vi "readblink.vi"() -> ()   [LabVIEW 2014]
uses:
  <vilib>/LabVIEW Interface for Arduino/Type Defs/Board Type.ctl
  <vilib>/addons/_Advanced Signal Processing/NI_AdvSigProcWA.lvlib
  <vilib>/LabVIEW Interface for Arduino/LabVIEW Interface for Arduino.lvlib
panel:
  in  "stop":bool
  out "Filtered Signal 4":waveform(dbl)(graph) caption="Filtered Signal"
  out "Boolean":bool
  out "Result":dynamicdata(graph)
  out "Filtered Signal 3":dynamicdata(graph) caption="Filtered Signal"
  out "Filtered Signal 2":dynamicdata(graph) caption="Filtered Signal"
  out "Filtered Signal":dynamicdata(graph)
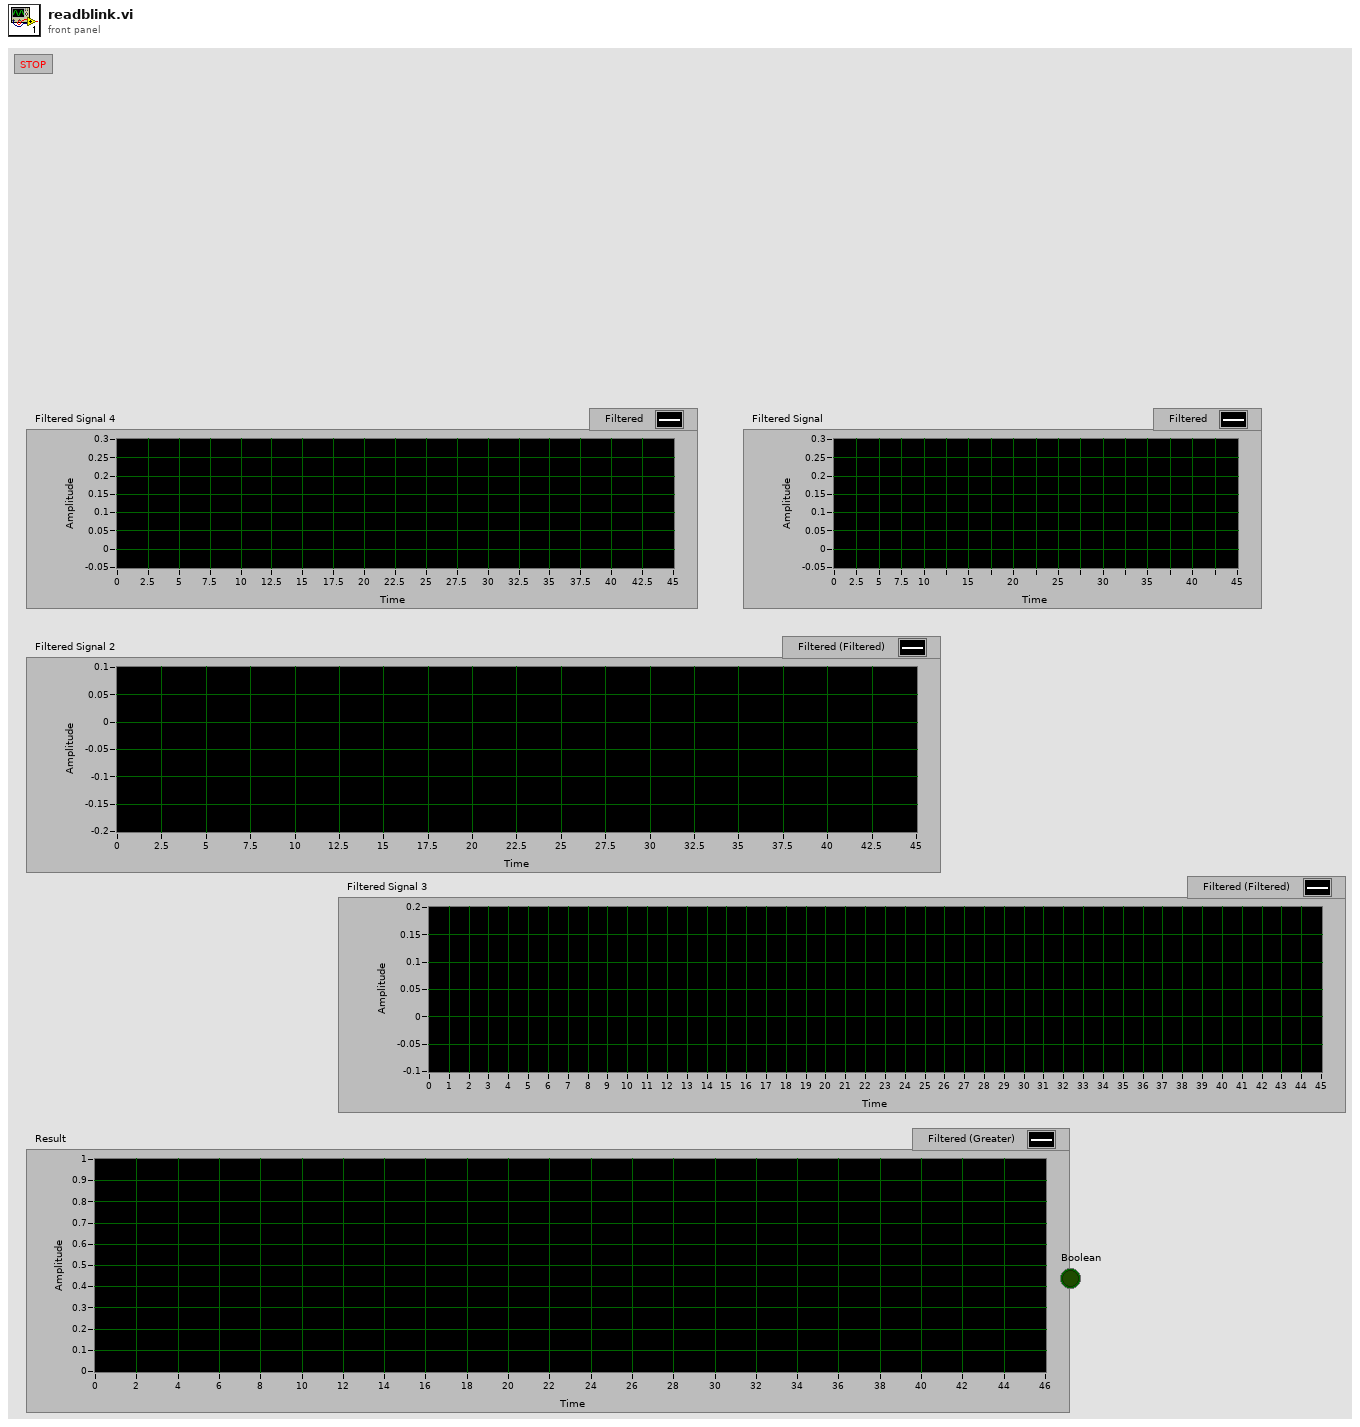
[diagram p1: front panel]
types:
  T1 = typedef "LabVIEW Interface for Arduino.lvlib/Board Type.ctl" = enum16{"Uno", "Dimuelanove w/Atmega 328", "Mega 2560"}
  T2 = typedef "LabVIEW Interface for Arduino.lvlib/Arduino Resource.ctl" = cluster{"VISA resource":refnum<visa-resource-name>, "Board Type":T1, "Connection Type":enum8{"USB / Serial"}, "Bytes Per Packet (15)":u8}
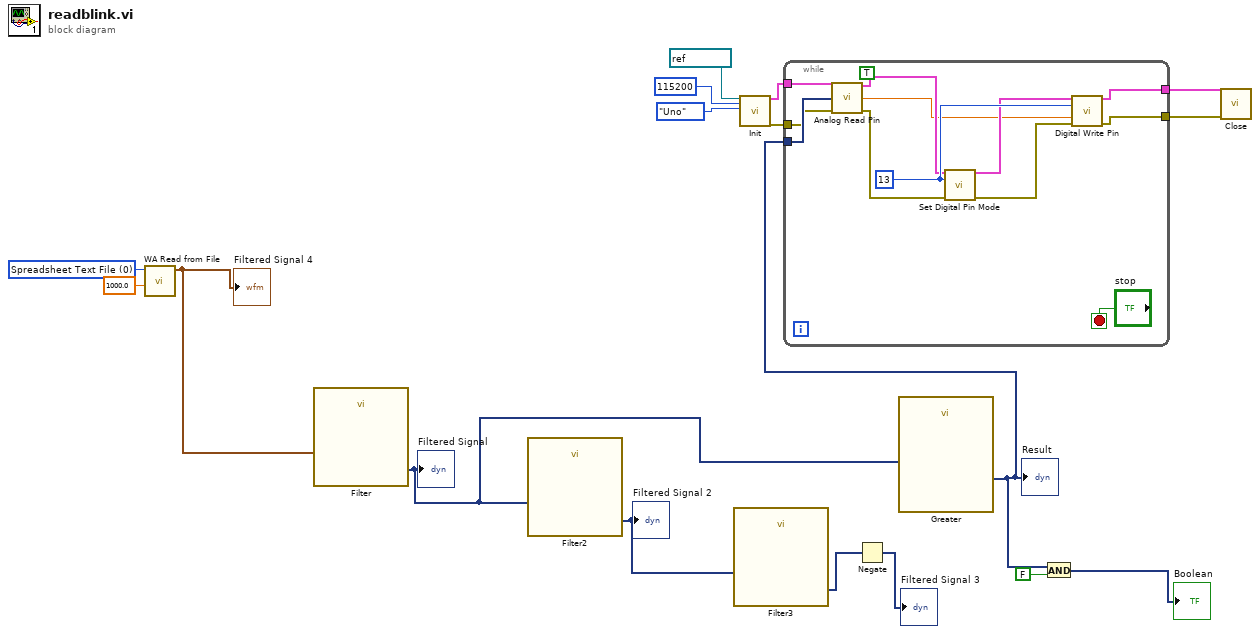
[diagram p0: block diagram]
diagram:
  w17 = u16 0 items=["Spreadsheet Text File", "Byte Stream File of SGL", "Byte Stream File of I16", "Waveforms Data File", "WAV File", "JPG File", "BMP File", "PNG File"] ("file type")
  n1 = call <vilib>:"WA Read from File.vi"("sampling rate"=1000.0, "file type"=w17) -> ("1D signal"=w9:waveform(dbl))  [unwired: 6 in, 3 out]
  "Filtered Signal 4" <- w9
  n2 = call "Filter"("Signal"=w9) -> ("Filtered Signal"=w10:dynamicdata)  [unwired: 9 in, 1 out]
  "Filtered Signal" <- w10
  n3 = call "Filter2"("Signal"=w10) -> ("Filtered Signal"=w15:dynamicdata)  [unwired: 9 in, 1 out]
  "Filtered Signal 2" <- w15
  n4 = call "Filter3"("Signal"=w15) -> ("Filtered Signal"=w14:dynamicdata)  [unwired: 9 in, 1 out]
  n5 = call <vilib>:"Init.vi"("VISA resource"=refnum<visa-resource-name> "COM4", "Baud Rate (115200)"=u32 115200, "Board Type (Uno)"=Board_Type."Uno") -> ("Arduino Resource"=w5:T2, "error out"=w2:errorcluster)  [unwired: 15 in]
  n6 = Negate(x=w14) -> (-x=→"Filtered Signal 3":dynamicdata)
  n7 = call "Greater"("Operand 1"=w10) -> ("Result"=w1:dynamicdata)  [unwired: 9 in, 1 out]
  "Result" <- w1
  n8 = while {
    tunnel: w5 -> [w26]
    tunnel: [w19] -> w4
    tunnel: [w22] -> w3
    tunnel: w2 -> [w27]
    tunnel: w1 -> [w28]
    stop <- "stop" stop-if-true
    (unwired) TRUE ("initialize")
    w25 = u8 13 ("Digital I/O Pin")
    n9 = call <vilib>:"Analog Read Pin.vi"("Arduino Resource"=w26, "Analog Input Pin (0)"=w28, "error in"=w27) -> ("Arduino Resource"=w24:T2, "Voltage"=w18:dbl, "error out"=w21:errorcluster)  [unwired: 10 in]
    n10 = call <vilib>:"Set Digital Pin Mode.vi"("Arduino Resource"=w24, "Digital I/O Pin"=w25, "error in"=w21) -> ("Arduino Resource"=w23:T2, "error out"=w20:errorcluster)  [unwired: 11 in]
    n11 = call <vilib>:"Digital Write Pin.vi"("Arduino Resource"=w23, "Digital I/O Pin (0)"=w25, "Value (0)"=w18, "error in"=w20) -> ("Arduino Resource"=w22:T2, "error out"=w19:errorcluster)  [unwired: 10 in]
  }
  n12 = And(x=w1, y=FALSE) -> (x .and. y?=→"Boolean":dynamicdata)
  n13 = call <vilib>:"Close.vi"("Arduino Resource"=w3, "error in"=w4) -> ()  [unwired: 13 in, 1 out]
